vi "SetSelectionColor.vi"(0 "reference in":refnum<class "DataGridView.lvclass">, 5 "BGColor":u32(colorbox), 7 "FGColor":u32(colorbox), 11 "error in (no error)":errorcluster) -> (4 "reference out":refnum<class "DataGridView.lvclass">, 15 "error out":errorcluster)   [LabVIEW 2018, in "DataGridView.lvclass"]
doc: "Sets the forecolor and the backcolor of the selected row"
uses:
  DataGridView.lvclass
  System.Windows.Forms
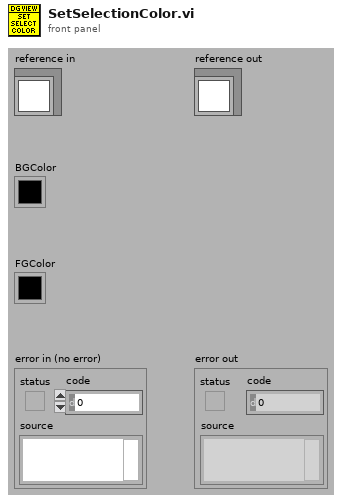
[diagram p1: front panel]
types:
  T1 = typedef "DataGridView.lvclass/ObjectAttributes.ctl" = cluster{"DataGridView":refnum<k24>, "SelectionChangedEvent":refnum<user-event>, "SelectionChanged callback ref":refnum<k27>, "LastSelectedRowIndex":i32}
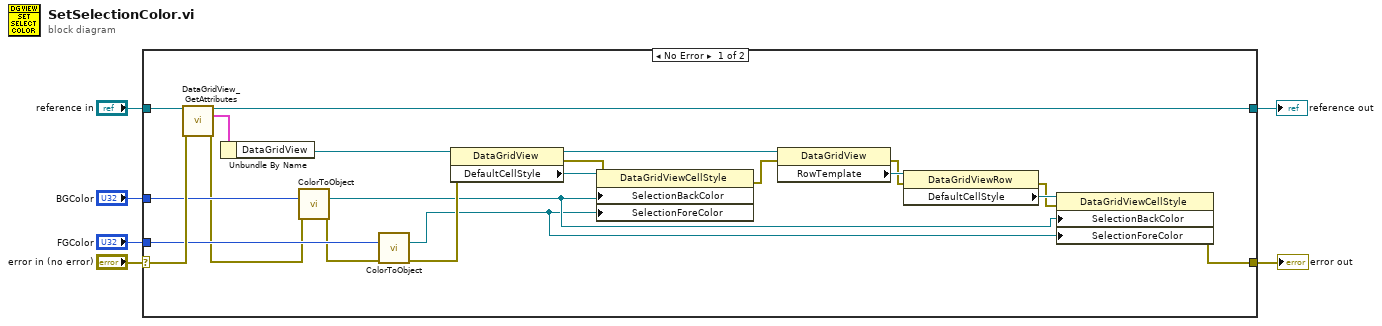
[diagram p0: block diagram]
diagram:
  n1 = case shown="No Error" "error in (no error)" {
    selector: "error in (no error)" -> [w27 w29]
    tunnel: [w7 w29] -> w5
    tunnel: [w16 w28] -> w3
    tunnel: "reference in" -> [w25 w28]
    tunnel: "BGColor" -> [w21 _]
    tunnel: "FGColor" -> [w20 _]
    frame No Error {
      n2 = call "DataGridView_GetAttributes.vi"("reference in"=w25, "error in (no error)"=w27) -> ("reference out"=w16:refnum<class "DataGridView.lvclass">, "Data"=w26:T1, "error out"=w19:errorcluster)  [unwired: 10 in, 1 out]
      n3 = Unbundle By Name(w26) -> ("DataGridView"=w24:refnum<k24>)
      n4 = call "ColorToObject.vi"("Color"=w21, "error in (no error)"=w19) -> (".Net Color"=w12:refnum<k24>, "error out"=w18:errorcluster)  [unwired: 12 in]
      n5 = call "ColorToObject.vi"("Color"=w20, "error in (no error)"=w18) -> (".Net Color"=w11:refnum<k24>, "error out"=w17:errorcluster)  [unwired: 12 in]
      n6 = property class="DataGridView"(reference=w24, error in=w17) -> (reference out=w15:refnum<k24>, error out=w22:errorcluster, "DefaultCellStyle"=w23:refnum<k24>)
      n7 = property class="DataGridViewCellStyle"(reference=w23, error in=w22, "SelectionBackColor"=w12, "SelectionForeColor"=w11) -> (error out=w8:errorcluster)  [unwired: 1 out]
      n8 = property class="DataGridView"(reference=w15, error in=w8) -> (error out=w10:errorcluster, "RowTemplate"=w14:refnum<k24>)  [unwired: 1 out]
      n9 = property class="DataGridViewRow"(reference=w14, error in=w10) -> (error out=w9:errorcluster, "DefaultCellStyle"=w13:refnum<k24>)  [unwired: 1 out]
      n10 = property class="DataGridViewCellStyle"(reference=w13, error in=w9, "SelectionBackColor"=w12, "SelectionForeColor"=w11) -> (error out=w7:errorcluster)  [unwired: 1 out]
    }
    frame Error {
    }
  }
  "error out" <- w5
  "reference out" <- w3
